vi "picture cutting.vi"(11 "length":i32) -> (0 "size X":i32, 1 "Y length":i32, 2 "select":T1, 3 "X length":i32, 4 "size Y":i32)   [LabVIEW 2014]
uses:
  <vilib>/picture/picture.llb/imagedata.ctl
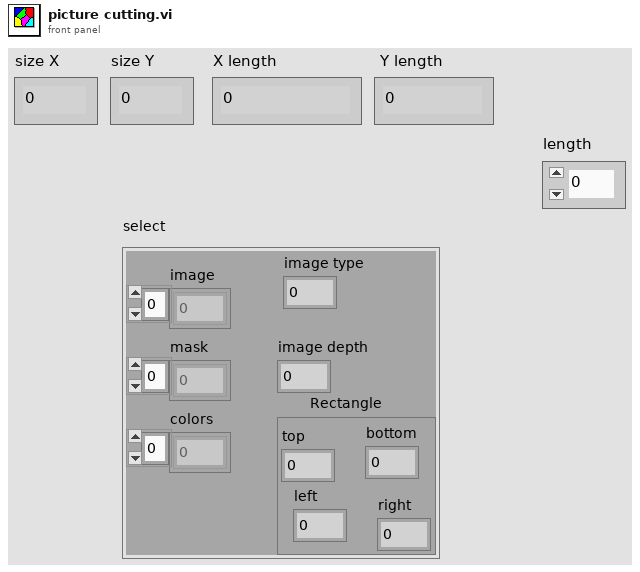
[diagram p1: front panel]
types:
  T1 = typedef "imagedata.ctl" = cluster{"image type":i32, "image depth":i32, "image":u8[], "mask":u8[], "colors":u32[], "Rectangle":cluster{"left":i16, "top":i16, "right":i16, "bottom":i16}}
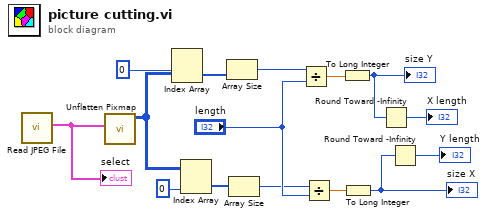
[diagram p0: block diagram]
diagram:
  n1 = call <vilib>:"Read JPEG File.vi"() -> ("image data"=w12:T1)  [unwired: 9 in, 2 out]
  "select" <- w12
  n2 = call <vilib>:"Unflatten Pixmap.vi"("image data"=w12) -> ("24-bit pixmap"=w5:u32[][])  [unwired: 4 in, 6 out]
  n3 = Index Array(array=w5, index (row)=0) -> (element=w8:u32[])  [unwired: 1 in]
  n4 = Index Array(array=w5, index (col)=0 ("disabled index (col)")) -> (element=w9:u32[])  [unwired: 1 in]
  n5 = Array Size(array=w8) -> (size(s)=w10:i32)
  n6 = Array Size(array=w9) -> (size(s)=w11:i32)
  n7 = Divide(x=w10, y="length") -> (x/y=w4:dbl)
  n8 = Divide(x=w11, y="length") -> (x/y=w2:dbl)
  n9 = To Long Integer(number=w4) -> (32bit integer=w3:i32)
  "size Y" <- w3
  n10 = To Long Integer(number=w2) -> (32bit integer=w1:i32)
  "size X" <- w1
  n11 = Round Toward -Infinity(1:w3) -> (0:→"X length":i32)
  n12 = Round Toward -Infinity(1:w1) -> (0:→"Y length":i32)
